vi "Multiplicate Mirrored inputs and outputs.vi"(6 "in 1":sgl, 10 "in 2":sgl) -> (7 "out":sgl)   [LabVIEW 2014]
doc: "Normal multiplication but inputs and outputs are mirrored."
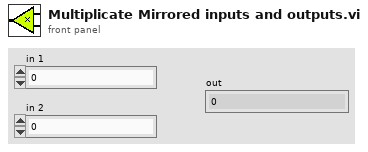
[diagram p1: front panel]
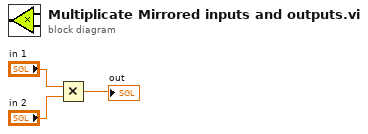
[diagram p0: block diagram]
diagram:
  n1 = Multiply(x="in 1", y="in 2") -> (x*y=→"out":sgl)
